vi "Get Real LUP Matrix.vi"(0 "LU Info":cluster{"LU":dbl[][], "Pivot":i32[]} {"LU" format="%.3f"}) -> (1 "L":T1, 2 "U":T1, 3 "P":i32[][](array[numeric]))   [LabVIEW 2018, in "NI_AALBase.lvlib"]
uses:
  <vilib>/Analysis/NI_AALBase.lvlib
  RealMatrix.ctl
  Array To Matrix - RA2.vi
  NI_Matrix.lvlib
panel:
  # "Get Real LUP Matrix"
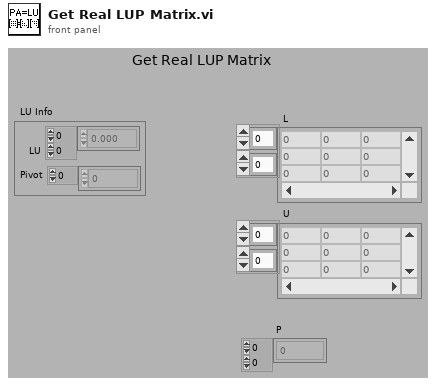
[diagram p1: front panel]
types:
  T1 = typedef "NI_Matrix.lvlib/RealMatrix.ctl" = dbl[][]
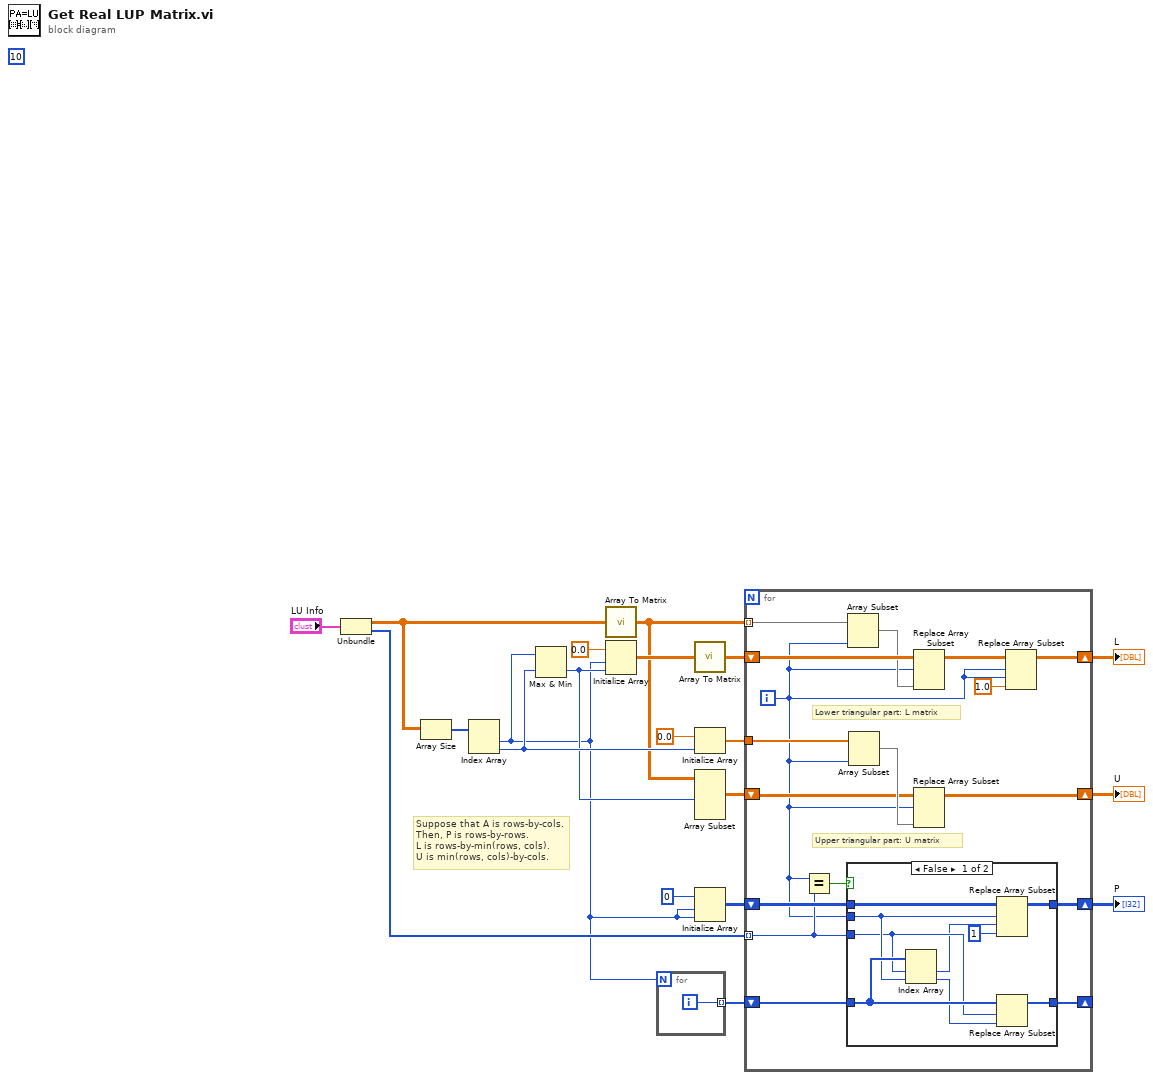
[diagram p0: block diagram]
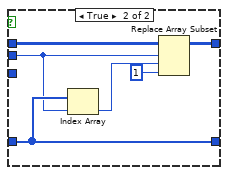
[diagram p2: hidden frame]
diagram:
  (unwired) 10
  # "Suppose that A is rows-by-cols.\nThen, P is rows-by-rows.\nL is rows-by-min(rows, cols).\nU is min(rows, cols)-by-cols."
  n1 = Unbundle("LU Info") -> ("LU"=w9:dbl[][], "Pivot"=w16:i32[])
  n2 = Array Size(array=w9) -> (size(s)=w15:i32[])
  n3 = Index Array(array=w15) -> (element #1=w6:i32, element #2=w11:i32)  [unwired: 2 in]
  n4 = Max & Min(x=w6, y=w11) -> (min(x,y)=w7:i32)  [unwired: 1 out]
  n5 = call-poly "Array To Matrix.vi"("Real 2D Array"=w9) -> ("Real Matrix"=w1:T1)
  n6 = Initialize Array(0.0 ("element"), w6, w7) -> (w13:dbl[][])
  n7 = for {
    N: w6 -> [_]
    tunnel: [w21] -> w17 mode=indexing
    i -> [w21]
  }
  n8 = call-poly "Array To Matrix.vi"("Real 2D Array"=w13) -> ("Real Matrix"=w12:T1)
  n9 = Initialize Array(0.0 ("element"), w11) -> (w20:dbl[])
  n10 = Array Subset(array=w1, length (row)=w7) -> (w8:T1)  [unwired: 3 in]
  n11 = Initialize Array(0, w6, w6) -> (w18:i32[][])
  n12 = for {
    tunnel: w1 -> [w37] mode=indexing
    shift-right: [w24] -> w5
    shift-left: w12 -> [w38]
    tunnel: w20 -> [w35]
    shift-right: [w32] -> w4
    shift-left: w8 -> [w33]
    shift-right: [w31] -> w3
    shift-left: w18 -> [w30]
    shift-right: [w28] -> _
    shift-left: w17 -> [w29]
    tunnel: w16 -> [w26] mode=indexing
    i -> [w23]
    # "Upper triangular part: U matrix"
    # "Lower triangular part: L matrix"
    n13 = Equal?(x=w23, y=w26) -> (x = y?=w27:bool)
    n14 = case shown="False" w27 {
      tunnel: w29 -> [w47 w50]
      tunnel: [w46 w50] -> w28
      tunnel: w26 -> [w41 _]
      tunnel: w23 -> [w42 w49]
      tunnel: w30 -> [w45 w53]
      tunnel: [w44 w52] -> w31
      frame False {
        n15 = Index Array(array=w47, index #1=w41, index #2=w42) -> (element #1=w39:i32, element #2=w40:i32)
        n16 = Replace Array Subset(array=w45, new element=1 ("new element/subarray"), index (row)=w42, index (col)=w39) -> (w44:i32[][])
        n17 = Replace Array Subset(array=w47, new element=w40, index=w41) -> (w46:i32[])
      }
      frame True {
        n18 = Index Array(array=w50, index=w49) -> (element=w48:i32)
        n19 = Replace Array Subset(array=w53, new element=1, index (row)=w49, index (col)=w48) -> (w52:i32[][])
      }
    }
    n20 = Array Subset(array=w37, length=w23) -> (w36:dbl[])  [unwired: 1 in]
    n21 = Array Subset(array=w35, length=w23) -> (w34:dbl[])  [unwired: 1 in]
    n22 = Replace Array Subset(array=w38, new element=w36, index (row)=w23) -> (w25:T1)  [unwired: 1 in]
    n23 = Replace Array Subset(array=w33, new element=w34, index (row)=w23) -> (w32:T1)  [unwired: 1 in]
    n24 = Replace Array Subset(array=w25, new element=1.0 ("new element/subarray"), index (row)=w23, index (col)=w23) -> (w24:T1)
  }
  "U" <- w4
  "L" <- w5
  "P" <- w3
